vi "Start.vi"(8 "error in (no error)":errorcluster, 11 "Vecto in":refnum<class "Vecto.lvclass">) -> (0 "error out":errorcluster, 3 "Vecto out":refnum<class "Vecto.lvclass">)   [LabVIEW 2020, in "Vecto.lvlib" / "Vecto.lvclass"]
uses:
  Vecto.lvclass
  Event Level.ctl
  Vecto.lvclass/Vecto.ctl
  EventLoggingService/EventLoggingService.lvclass/EventLoggingService.ctl
  <vilib>/Utility/error.llb/Error Cluster From Error Code.vi
  EventLogHandler/EventLogHandler.lvclass
  Vecto.lvlib
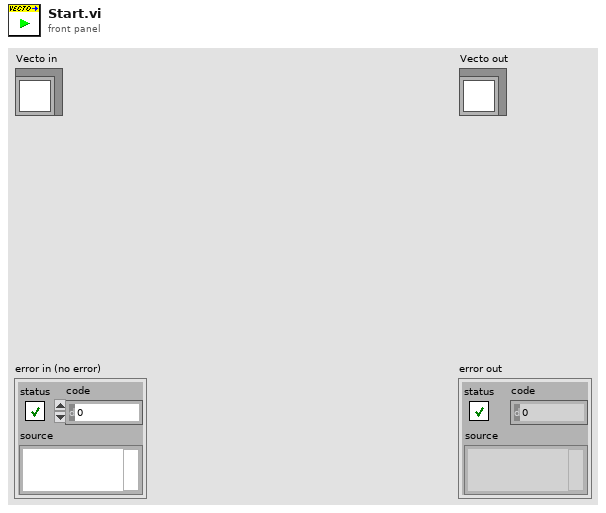
[diagram p1: front panel]
types:
  T1 = typedef "Vecto.lvlib/Event Level.ctl" = enum16{"Debug", "Info", "Warning", "Error"}
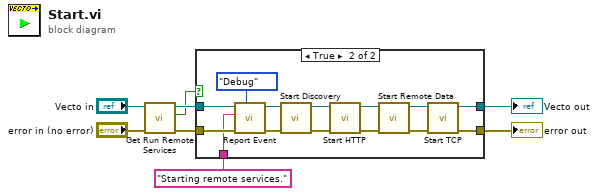
[diagram p0: block diagram]
diagram:
  n1 = call "Get Run Remote Services.vi"("error in (no error)"="error in (no error)", "Vecto in"="Vecto in") -> ("error out"=w5:errorcluster, "Run Remote Services"=w2:bool, "Vecto out"=w3:refnum<class "Vecto.lvclass">)  [unwired: 7 in]
  n2 = case shown="True" w2 {
    tunnel: [w9 w18] -> w7
    tunnel: [w10 w16] -> w6
    tunnel: w5 -> [w9 w21]
    tunnel: w3 -> [w10 w14]
    tunnel: "Starting remote services." -> [_ w12]
    frame False {
    }
    frame True {
      n3 = call "Report Event.vi"("Event Level (Info)"=Event_Level."Debug", "error in (no error)"=w21, "Message"=w12, "Vecto in"=w14) -> ("error out"=w15:errorcluster, "Vecto out"=w13:refnum<class "Vecto.lvclass">)  [unwired: 6 in]
      n4 = call "Start Discovery.vi"("error in (no error)"=w15, "Vecto in"=w13) -> ("error out"=w23:errorcluster, "Vecto out"=w22:refnum<class "Vecto.lvclass">)  [unwired: 8 in]
      n5 = call "Start HTTP.vi"("error in (no error)"=w23, "Vecto in"=w22) -> ("error out"=w24:errorcluster, "Vecto out"=w19:refnum<class "Vecto.lvclass">)  [unwired: 8 in]
      n6 = call "Start Remote Data.vi"("error in (no error)"=w24, "Vecto in"=w19) -> ("error out"=w20:errorcluster, "Vecto out"=w17:refnum<class "Vecto.lvclass">)  [unwired: 8 in]
      n7 = call "Start TCP.vi"("error in (no error)"=w20, "Vecto in"=w17) -> ("error out"=w18:errorcluster, "Vecto out"=w16:refnum<class "Vecto.lvclass">)  [unwired: 8 in]
    }
  }
  "error out" <- w7
  "Vecto out" <- w6
